vi "ROI_to_norm_ROI_Convertor.vi"(10 "Experiment folder path":path, 11 "XYZ Coordinates":T1[](array[typedef]) {"ROI group ID" format="%#_6f"; "Laser Power (%)" format="%#_6f"; "Zoom" format="%#_6f"; "Frame Size" format="%#_6f"; "Number of lines" format="%#_6f"; "Composite ID" format="%#_6f"; "Angle (deg)" format="%#_6f"; "ROI Time (ns)" format="%#_6f"; "ROI ID" format="%#_6f"; "Pixels in ROI" format="%#_6f"; "ROI index" format="%#_6f"; "Z stop" format="%#_6f"; "Y stop" format="%#_6f"; "X stop" format="%#_6f"; "Z start" format="%#_6f"; "X start" format="%#_6f"; "Y start" format="%#_6f"}) -> (3 "norm_XYZ_Coordinates":T1[](array[typedef]) {"ROI group ID" format="%#_6f"; "Laser Power (%)" format="%#_6f"; "Zoom" format="%#_6f"; "Frame Size" format="%#_6f"; "Number of lines" format="%#_6f"; "Composite ID" format="%#_6f"; "Angle (deg)" format="%#_6f"; "ROI Time (ns)" format="%#_6f"; "ROI ID" format="%#_6f"; "Pixels in ROI" format="%#_6f"; "ROI index" format="%#_6f"; "Z stop" format="%#_6f"; "Y stop" format="%#_6f"; "X stop" format="%#_6f"; "Z start" format="%#_6f"; "X start" format="%#_6f"; "Y start" format="%#_6f"})   [LabVIEW 2013]
uses:
  Visualisation/Functional Imaging Viewer/Typedefs/ROI parameters data type.ctl
  Global Variables/gl_UI Ctrl Refs.vi
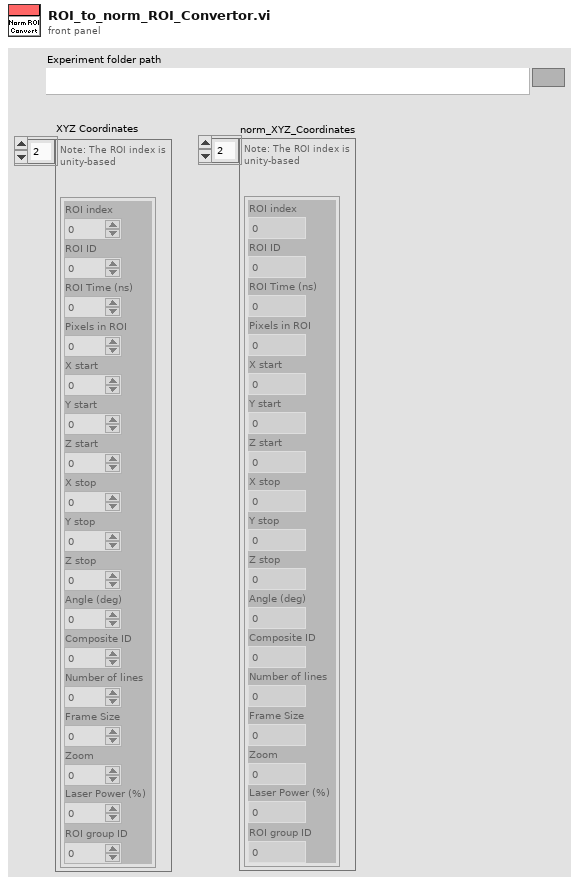
[diagram p1: front panel]
types:
  T1 = typedef "ROI parameters data type.ctl" = cluster{"ROI index":dbl, "ROI ID":dbl, "ROI Time (ns)":dbl, "Pixels in ROI":dbl, "X start":dbl, "Y start":dbl, "Z start":dbl, "X stop":dbl, "Y stop":dbl, "Z stop":dbl, "Angle (deg)":dbl, "Composite ID":dbl, "Number of lines":dbl, "Frame Size":dbl, "Zoom":dbl, "Laser Power (%)":dbl, "ROI group ID":dbl}
  T2 = typedef "Image Type" = u32
  T3 = typedef "UI ctrl refs cluster.ctl" = cluster{"Top level VI path":path, "Top level VI ref":refnum<vi>, "User menu ref":refnum<k9>, "Sub Panel control":refnum<vi>, "Imaging Param Tab":refnum<vi>, "Occurrence-Start drivers":refnum<k4>, "Occurrence-Speed logging initialised":refnum<k4>, "Occurrence-XYZ stage initialised":refnum<k4>, "Exit button":refnum<vi>, "Status ind":refnum<vi>, "Return to Origin":refnum<vi>, "Speed Logging":refnum<vi>, "Time Lapse":refnum<vi>, "Live Imaging":refnum<vi>, "AOL Z Stack":refnum<vi>, "Motor Z Stack":refnum<vi>, "Funct Acq button":refnum<vi>, "Hard Shutter":refnum<vi>, "Virtual Shutter":refnum<vi>, "Laser Power":refnum<vi>, "AOL Mode":refnum<vi>, "Frame Size":refnum<vi>, "Field of View":refnum<vi>, "Dwell Time":refnum<vi>, "Zoom":refnum<vi>, "AOL Z":refnum<vi>, "Objective":refnum<vi>, "Axis":refnum<vi>, "Paths & Names":refnum<vi>, "Experiment folder path (ind.)":refnum<vi>, "Last State (Ind.)":refnum<vi>, "Laser wavelength ind (nm)":refnum<vi>, "Averages":refnum<vi>, "Angle (degrees)":refnum<vi>, "X centre":refnum<vi>, "Y centre":refnum<vi>, "Plane Mode":refnum<vi>, "# Planes":refnum<vi>, "Z Start":refnum<vi>, "Z Stop":refnum<vi>, "Z Step":refnum<vi>, "PMT 1":refnum<vi>, "PMT 2":refnum<vi>, "Stage XYZ Position":refnum<vi>, "Pockels@Z Start":refnum<vi>, "Pockels@Z Stop":refnum<vi>, "Obtain Z Start":refnum<vi>, "Obtain Z Stop":refnum<vi>, "Live stim.trig.period":refnum<vi>, "Live stim.trig.enable":refnum<vi>, "Funct. Acq. Pockels Modulation":refnum<vi>, "Enable Video Recording":refnum<vi>, "Video Record-Live Imaging":refnum<vi>, "Video Record-Funct acq":refnum<vi>, "AOL Z-stack Chirps Ready (ind)":refnum<vi>, "Center freq ind (nm)":refnum<vi>, "Logging queue (ind)":refnum<vi>, "Back aperture power (ind.)":refnum<vi>, "Power after objective (ind.)":refnum<vi>, "Switch user":refnum<vi>}
  T4 = typedef "Fixed strings.ctl" = cluster{"ROI file name":string, "Normalised ROI file name":string, "Zplane Pockels values file name":string, "Functional data folder name":string, "Experiment Header file name":string, "Z-stack images folder name":string, "Groups setup rel. path":string, "Groups text file rel. path":string, "TDMS files folder name (F.img)":string, "TDMS files folder name (V.acq)":string, "TDMS files folder name (Pl.acq)":string, "Cycle rel times sequence file":string, "Dynamically called VIs folder name":string, "Time Series folder base name":string}
  T5 = typedef "IMAQ Image.ctl" = refnum<image>
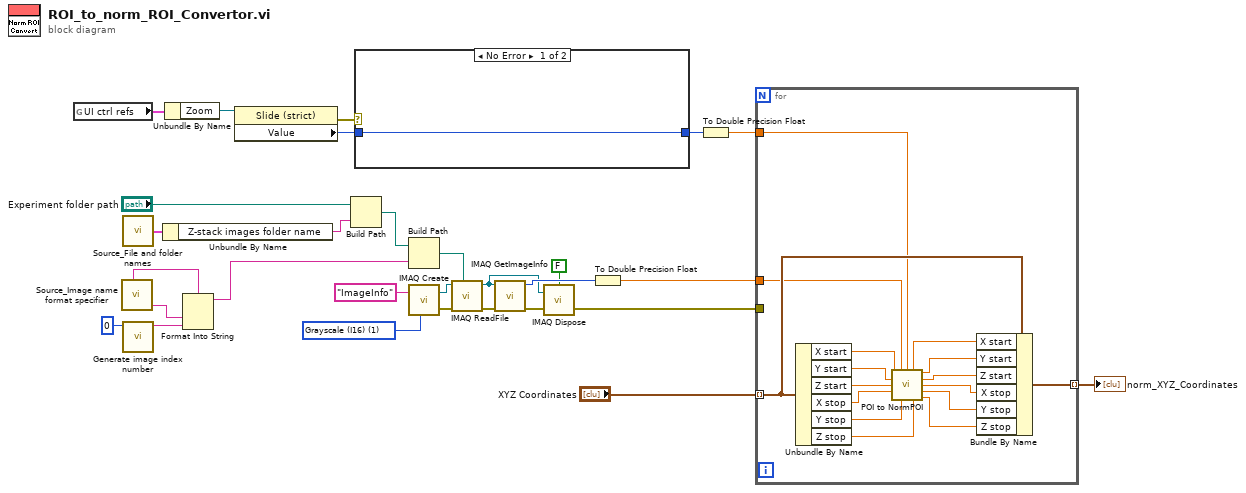
[diagram p0: block diagram]
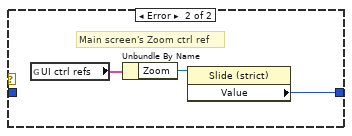
[diagram p2: hidden frame]
diagram:
  w27 = T2 1 items=["Grayscale (U8)", "Grayscale (I16)", "Grayscale (SGL)", "Complex (CSG)", "RGB (U32)", "HSL (U32)", "RGB (U64)", "Grayscale (U16)"] ("Image Type")
  n1 = global read "gl_UI Ctrl Refs.vi" "UI ctrl refs"() -> (w7:T3)
  n2 = call "Source_Image name format specifier.vi"() -> ("Z-Stack Image name format specifier"=w12:string, "Green channel name"=w8:string)  [unwired: 5 in, 1 out]
  n3 = call "Source_File and folder names.vi"() -> ("Fixed strings"=w16:T4)  [unwired: 1 in]
  n4 = call "Generate image index number.vi"("FOR loop iteration or existing number of files"=0) -> ("Number in string representation (padded with zeroes)"=w10:string)  [unwired: 10 in]
  n5 = Unbundle By Name(w16) -> ("Z-stack images folder name"=w15:string)
  n6 = Unbundle By Name(w7) -> ("Zoom"=w6:refnum<vi>)
  n7 = Format Into String(format string=w12, w8, w10) -> (resulting string=w9:string)  [unwired: 2 in, 1 out]
  n8 = property class="Slide (strict)"(reference=w6) -> (error out=w4:errorcluster, "Value"=w2:i8)  [unwired: 1 in, 1 out]
  n9 = Build Path(base path="Experiment folder path", name or relative path=w15) -> (appended path=w18:path)
  n10 = case shown="No Error" w4 {
    tunnel: w2 -> [w30 _]
    tunnel: [w30 w31] -> w3
    frame No Error {
    }
    frame Error {
      # "Main screen's Zoom ctrl ref"
      n11 = global read "gl_UI Ctrl Refs.vi" "UI ctrl refs"() -> (w33:T3)
      n12 = Unbundle By Name(w33) -> ("Zoom"=w32:refnum<vi>)
      n13 = property class="Slide (strict)"(reference=w32) -> ("Value"=w31:i8)  [unwired: 1 in, 2 out]
    }
  }
  n14 = Build Path(base path=w18, name or relative path=w9) -> (appended path=w24:path)
  n15 = call "IMAQ Create"("Image Name"="ImageInfo", "Image Type"=w27) -> ("New Image"=w25:T5, "error out"=w23:errorcluster)  [unwired: 3 in]
  n16 = call "IMAQ ReadFile"("File Path"=w24, "error in (no error)"=w23, "Image"=w25) -> ("error out"=w22:errorcluster, "Image Out"=w20:T5)  [unwired: 4 in, 3 out]
  n17 = call "IMAQ GetImageInfo"("error in (no error)"=w22, "Image"=w20) -> ("error out"=w21:errorcluster, "X Resolution"=w28:i32)  [unwired: 2 in, 6 out]
  n18 = call "IMAQ Dispose"("All Images? (No)"=FALSE, "Image"=w20, "error in (no error)"=w21) -> ("error out"=w13:errorcluster)  [unwired: 3 in]
  n19 = To Double Precision Float(number=w28) -> (double precision float=w5:dbl)
  n20 = To Double Precision Float(number=w3) -> (double precision float=w1:dbl)
  n21 = for {
    tunnel: "XYZ Coordinates" -> [w36] mode=indexing
    tunnel: [w46] -> w14 mode=indexing
    tunnel: w5 -> [w35]
    tunnel: w13 -> [_]
    tunnel: w1 -> [w34]
    n22 = Unbundle By Name(w36) -> ("X start"=w49:dbl, "Y start"=w48:dbl, "Z start"=w47:dbl, "X stop"=w42:dbl, "Y stop"=w41:dbl, "Z stop"=w40:dbl)
    n23 = call "POI to NormPOI.vi"("X start"=w49, "FrameSize"=w35, "Zoom"=w34, "Y start"=w48, "Z start"=w47, "X stop"=w42, "Y stop"=w41, "Z stop"=w40) -> ("Norm XStart"=w44:dbl, "Norm YStart"=w43:dbl, "Norm ZStart"=w45:dbl, "Norm XStop"=w39:dbl, "Norm YStop"=w38:dbl, "Norm ZStop"=w37:dbl)  [unwired: 2 in]
    n24 = Bundle By Name(cluster=w36, "X start"=w44, "Y start"=w43, "Z start"=w45, "X stop"=w39, "Y stop"=w38, "Z stop"=w37) -> (w46:T1)
  }
  "norm_XYZ_Coordinates" <- w14
